vi "TypeDescriptor_GetPString.vi"(10 "offset (0)":i32, 11 "I16 String Descriptor":i16[](array[numeric])) -> (3 "String":string)   [LabVIEW 2013, in "OpenDescriptor.lvlib"]
uses:
  OpenDescriptor.lvlib
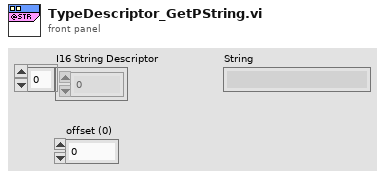
[diagram p1: front panel]
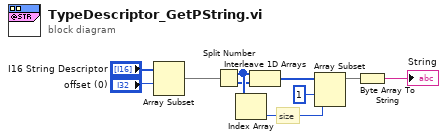
[diagram p0: block diagram]
diagram:
  # "size"
  n1 = Array Subset(array="I16 String Descriptor", index="offset (0)") -> (w2:i16[])  [unwired: 1 in]
  n2 = Split Number(x=w2) -> (hi(x)=w7:u8[], lo(x)=w4:u8[])
  n3 = Index Array(array=w7) -> (element=w8:u8)  [unwired: 1 in]
  n4 = Interleave 1D Arrays(w7, w4) -> (w5:u8[])
  n5 = Array Subset(array=w5, index=1, length=w8) -> (w9:u8[])
  n6 = Byte Array To String(unsigned byte array=w9) -> (string=→"String":string)
